vi "Agilent 2000 3000 X-Series Ripple Power Analysis.vi"() -> ()   [LabVIEW 2015]
doc: "This example shows how to apply a Ripple Power Analysis and read the measurement data. \n\n<B>Note:</B> This example is only applicable when the DSOX3PWR power measurements and analysis application is licensed and enabled."
uses:
  <instrlib>/Agilent 2000 3000 X-Series/Public/Data/Read Measurement (Ripple Power Analysis).vi
  <instrlib>/Agilent 2000 3000 X-Series/Agilent 2000 3000 X-Series.lvlib
panel:
  out "Ripple Measurement Result":dbl
  in  "Measurement Source 2 (1: Channel 2)":i32(ring)=1 items=["Channel 1", "Channel 2", "Channel 3", "Channel 4", "Math", "Waveform Memory 1", "Waveform Memory 2"]
  in  "Measurement Source 1 (0: Channel 1)":i32(ring) items=["Channel 1", "Channel 2", "Channel 3", "Channel 4", "Math", "Waveform Memory 1", "Waveform Memory 2", "External", "D0", "D1", "D2", "D3", "D4", "D5", "D6", "D7", "D8", "D9", "D10", "D11", "D12", "D13", "D14", "D15"]
  in  "VISA resource name":refnum<visa-resource-name>
  # "(c) 2011-2016 National Instruments.  ALL RIGHTS RESERVED."
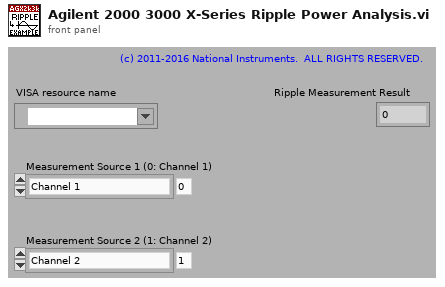
[diagram p1: front panel]
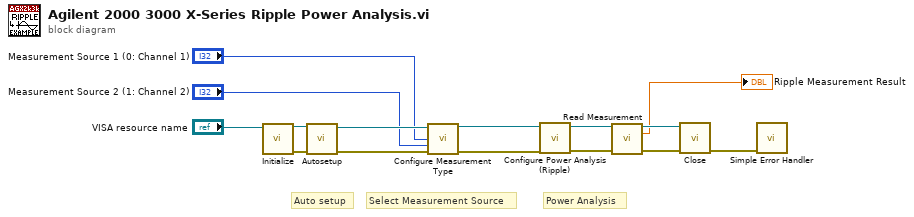
[diagram p0: block diagram]
diagram:
  # "Power Analysis"
  # "Select Measurement Source"
  # "Auto setup"
  n1 = call <instrlib>:"Initialize.vi"("VISA resource name"="VISA resource name") -> ("error out"=w13:errorcluster, "VISA resource name out"=w12:refnum<visa-resource-name>)  [unwired: 4 in, 5 out]
  n2 = call <instrlib>:"Autosetup.vi"("error in (no error)"=w13, "VISA resource name"=w12) -> ("error out"=w10:errorcluster, "VISA resource name out"=w11:refnum<visa-resource-name>)  [unwired: 4 in, 4 out]
  n3 = call <instrlib>:"Configure Measurement Type.vi"("VISA resource name"=w11, "Measurement Source 1 (0: Channel 1)"="Measurement Source 1 (0: Channel 1)", "Measurement Source 2 (1: Channel 2)"="Measurement Source 2 (1: Channel 2)", "error in (no error)"=w10) -> ("VISA resource name out"=w4:refnum<visa-resource-name>, "error out"=w2:errorcluster)  [unwired: 3 in, 7 out]
  n4 = call <instrlib>:"Configure Power Analysis (Ripple).vi"("error in (no error)"=w2, "VISA resource name"=w4) -> ("error out"=w1:errorcluster, "VISA resource name out"=w3:refnum<visa-resource-name>)  [unwired: 8 out]
  n5 = call-poly <instrlib>:"Read Measurement.vi"("VISA resource name"=w3, "error in (no error)"=w1) -> ("VISA resource name out"=w7:refnum<visa-resource-name>, "Ripple Measurement"=→"Ripple Measurement Result":dbl, "error out"=w6:errorcluster)  [unwired: 11 out]
  n6 = call <instrlib>:"Close.vi"("error in (no error)"=w6, "VISA resource name"=w7) -> ("error out"=w15:errorcluster)  [unwired: 9 out]
  n7 = call <vilib>:"Simple Error Handler.vi"("error in (no error)"=w15) -> ()  [unwired: 1 in, 8 out]
